vi "ExtractControlRefRecursive.vi"(6 "HierarchyLevel":i32, 8 "error in (no error)":errorcluster, 10 "ParentName":string, 11 "Controls[]":refnum<vi>[](array[refnum])) -> (0 "error out":errorcluster, 3 "Array":T1[](array[typedef]))   [LabVIEW 2020, in "ContextHelpEditor.lvlib"]
uses:
  ContextHelpEditor.lvlib
  ControlRef--cluster.ctl
  <vilib>/picture/picture.llb/imagedata.ctl
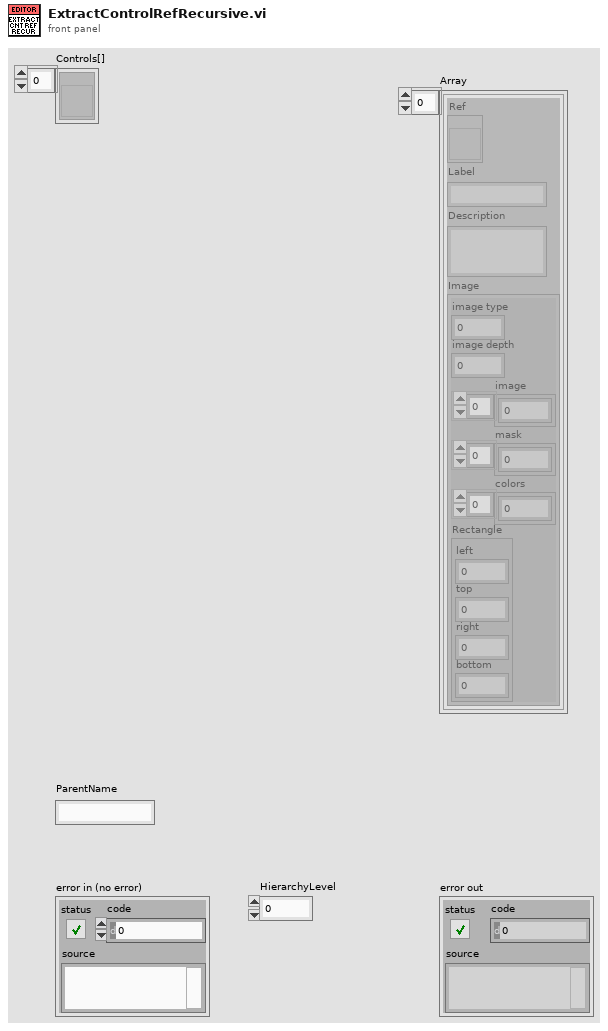
[diagram p1: front panel]
types:
  T1 = typedef "ContextHelpEditor.lvlib/ControlRef--cluster.ctl" = cluster{"Ref":refnum<vi>, "Label":string, "Description":string, "Image":T2}
  T2 = typedef "imagedata.ctl" = cluster{"image type":i32, "image depth":i32, "image":u8[], "mask":u8[], "colors":u32[], "Rectangle":cluster{"left":i16, "top":i16, "right":i16, "bottom":i16}}
  T3 = enum32{"not a typedef", "typedef", "strict typedef", "class private data"}
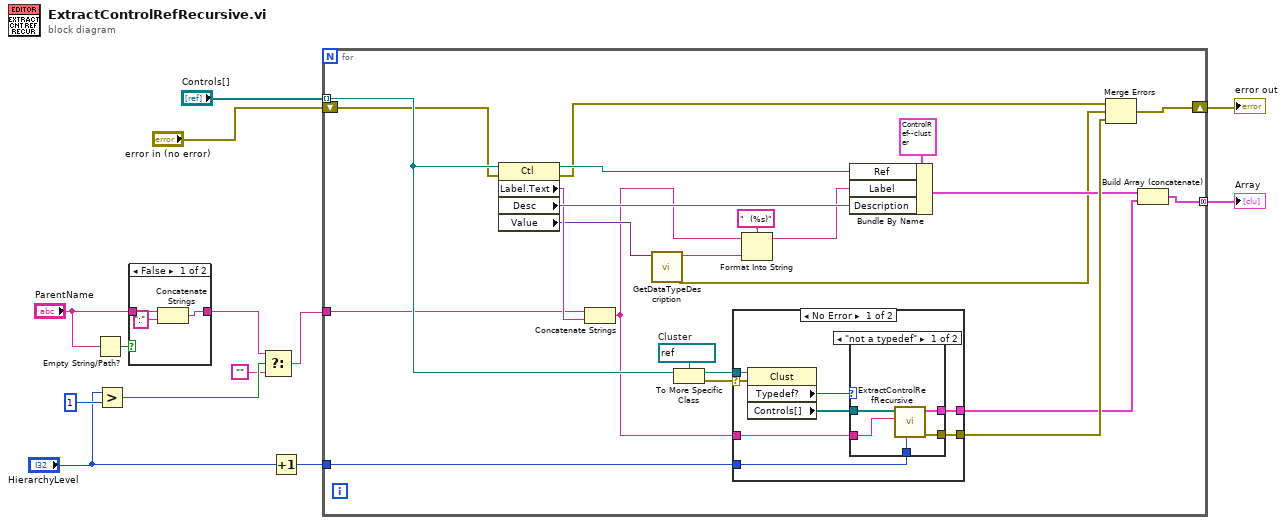
[diagram p0: block diagram]
diagram:
  n1 = Empty String/Path?(string/path="ParentName") -> (empty?=w5:bool)
  n2 = Greater?(x="HierarchyLevel", y=1) -> (0:w4:bool)
  n3 = case shown="False" w5 {
    tunnel: "ParentName" -> [w16 w17]
    tunnel: [w14 w17] -> w3
    frame False {
      n4 = Concatenate Strings(w16, ":" ("string")) -> (w14:string)
    }
    frame True {
    }
  }
  n5 = Select(t=w3, s=w4, f="") -> (s? t:f=w2:string)
  n6 = Increment(x="HierarchyLevel") -> (x+1=w6:i32)
  n7 = for {
    tunnel: "Controls[]" -> [w40] mode=indexing
    tunnel: [w39] -> w12 mode=concatenating
    shift-right: [w37] -> w13
    shift-left: "error in (no error)" -> [w38]
    tunnel: w2 -> [w25]
    tunnel: w6 -> [w24]
    w32 = refnum<vi> refnum  # Cluster
    n8 = property class="Ctl"(reference=w40, error in=w38) -> (reference out=w35:refnum<vi>, error out=w33:errorcluster, "Label.Text"=w26:string, "Desc"=w34:string, "Value"=w23:variant)
    n9 = Concatenate Strings(w25, w26) -> (w20:string)
    n10 = call "GetDataTypeDescription.vi"("Value"=w23) -> ("error out"=w22:errorcluster, "Datatype Description"=w21:string)  [unwired: 9 in]
    n11 = To More Specific Class(target class=w32, reference=w40) -> (specific class reference=w31:refnum<vi>, error out=w30:errorcluster)  [unwired: 1 in]
    n12 = case shown="No Error" w30 {
      selector: w30 -> [w47 _]
      tunnel: w31 -> [w48 _]
      tunnel: w20 -> [w44 _]
      tunnel: [w43 _] -> w27
      tunnel: [w42 _] -> w29
      tunnel: w24 -> [w41 _]
      frame No Error {
        n13 = property class="Clust"(reference=w48, error in=w47) -> ("Typedef?"=w46:T3, "Controls[]"=w45:refnum<vi>[])  [unwired: 2 out]
        n14 = case shown="\"not a typedef\"" w46 {
          tunnel: w45 -> [w53 _]
          tunnel: w44 -> [w52 _]
          tunnel: [w51 _] -> w43
          tunnel: [w50 _] -> w42
          tunnel: w41 -> [w49 _]
          frame "not a typedef" {
            n15 = call "ExtractControlRefRecursive.vi"("HierarchyLevel"=w49, "ParentName"=w52, "Controls[]"=w53) -> ("error out"=w50:errorcluster, "Array"=w51:T1[])  [unwired: 7 in]
          }
          frame Default {
          }
        }
      }
      frame Error {
      }
    }
    n16 = Format Into String(format string="  (%s)", initial string=w20, w21) -> (resulting string=w19:string)  [unwired: 1 in, 1 out]
    n17 = Bundle By Name(cluster=T1 {"Ref"=refnum, "Label"="", "Description"="", "Image"={"image type"=0, "image depth"=0, "image"=[], "mask"=[], "colors"=[], "Rectangle"={"left"=0, "top"=0, "right"=0, "bottom"=0}}} ("ControlRef"), "Ref"=w35, "Label"=w19, "Description"=w34) -> (w28:T1)
    n18 = Merge Errors(w33, w22, w29) -> (w37:errorcluster)
    n19 = Build Array (concatenate)(w28, w27) -> (w39:T1[])
  }
  "error out" <- w13
  "Array" <- w12
